vi "FPGA Definite Time Delay.vi"(0 "pick-up signal? (F)":bool, 1 "number of channels":T2=1 items=["1"=1, "2"=2, "3"=3, "4"=4, "5"=5, "6"=6, "7"=7, "8"=8, "9"=9, "10"=10, "11"=11, "12"=12, "13"=13, "14"=14, "15"=15, "16"=16], 5 "time delay settings":T1, 9 "input valid? (T)":bool=TRUE, 13 "instantaneous reset after tripping? (F)":bool) -> (4 "trip signal?":bool)   [LabVIEW 2013, in "NI_EP_Protection_FPGA.lvlib"]
doc: "Delays for the time interval that you specify in <B>time delay settings</B>, which includes the operate time and the reset time. Use this VI to build a protection relay with definite time delay characteristics, such as a 27 undervoltage relay, 50 instantaneous overcurrent relay, 59 overvoltage relay, and 81 frequency relay. You can compensate for the processing delay of the input energizing quantity to achieve higher operate time accuracy."
uses:
  <vilib>/addons/Electrical Power/Protection/NI_EP_Protection_FPGA.lvlib
  <vilib>/addons/Electrical Power/PQ/Resampling/FPGA/subVIs/fpga_NofCH.ctl
  <vilib>/addons/Electrical Power/Protection/Definite Time Delay/subVIs/fpga_Time Delay Cfg.ctl
  <vilib>/addons/Electrical Power/Protection/Definite Time Delay/subVIs/fpga_Feedback Var.ctl
  <vilib>/addons/Electrical Power/Protection/Definite Time Delay/subVIs/fpga_Timer Feedback Var.ctl
  <vilib>/addons/Electrical Power/Protection/Definite Time Delay/subVIs/fpga_State.ctl
  <vilib>/addons/Electrical Power/PQ/Resampling/NI_EP_Resample_FPGA.lvlib
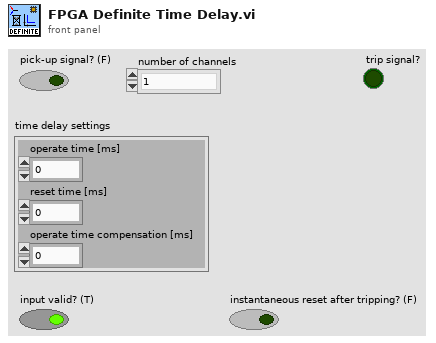
[diagram p1: front panel]
types:
  T1 = typedef "NI_EP_Protection_FPGA.lvlib/fpga_Time Delay Cfg.ctl" = cluster{"operate time [ms]":u32, "reset time [ms]":u32, "operate time compensation [ms]":u32}
  T2 = typedef "NI_EP_Resample_FPGA.lvlib/fpga_NofCH.ctl" = u8
  T3 = typedef "NI_EP_Protection_FPGA.lvlib/fpga_Feedback Var.ctl" = cluster{"timer":T4, "status":T5, "trip signal?":bool}
  T4 = typedef "NI_EP_Protection_FPGA.lvlib/fpga_Timer Feedback Var.ctl" = cluster{"time elapsed":u32, "start time of trip counting":u32, "start time of reseting":u32}
  T5 = typedef "NI_EP_Protection_FPGA.lvlib/fpga_State.ctl" = enum16{"Idle", "Trip Counting", "Tripped", "Reset Counting"}
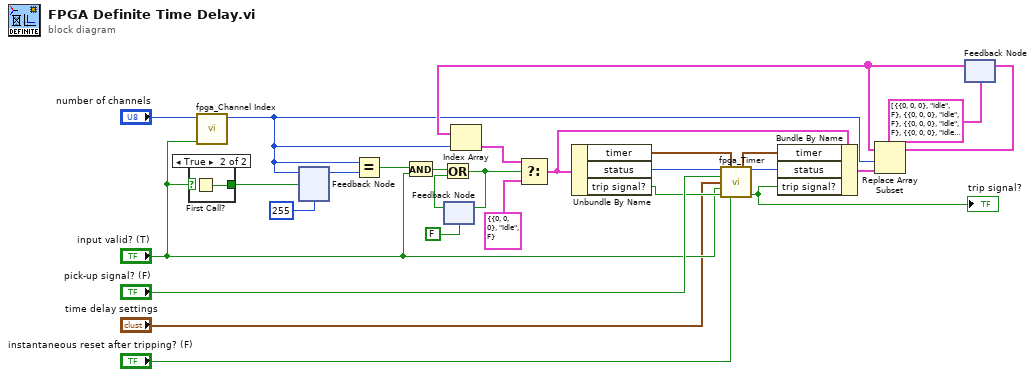
[diagram p0: block diagram]
diagram:
  n1 = case shown="True" "input valid? (T)" {
    selector: "input valid? (T)" -> [w28 _]
    tunnel: [w28 w29] -> w8
    frame False {
    }
    frame True {
      n2 = First Call?() -> (First Call?: T/F=w29:bool)
    }
  }
  n3 = call <vilib>:"fpga_Channel Index.vi"("input valid? (T)"="input valid? (T)", "number of channels"="number of channels") -> ("channel index"=w4:u8)  [unwired: 9 in]
  n4 = feedback #1(u8 255 ("channel index")) -> (w7:u8)
  n5 = feedback-in #1(w4, w8) -> ()
  n6 = Equal?(x=w4, y=w7) -> (x = y?=w11:bool)
  n7 = And(x=w11, y="input valid? (T)") -> (x .and. y?=w10:bool)
  n8 = feedback #2(FALSE) -> (w6:bool)
  n9 = Or(x=w10, y=w6) -> (x .or. y?=w19:bool)
  n10 = feedback-in #2(w19) -> ()
  n11 = feedback #3(T3[] [{"timer"={"time elapsed"=0, "start time of trip counting"=0, "start time of reseting"=0}, "status"=enum."Idle", "trip signal?"=FALSE}, {"timer"={"time elapsed"=0, "start time of trip counting"=0, "start time of reseting"=0}, "status"=enum."Idle", "trip signal?"=FALSE}, {"timer"={"time elapsed"=0, "start time of trip counting"=0, "start time of reseting"=0}, "status"=enum."Idle", "trip signal?"=FALSE}, {"timer"={"time elapsed"=0, "start time of trip counting"=0, "start time of reseting"=0}, "status"=enum."Idle", "trip signal?"=FALSE}, {"timer"={"time elapsed"=0, "start time of trip counting"=0, "start time of reseting"=0}, "status"=enum."Idle", "trip signal?"=FALSE}, {"timer"={"time elapsed"=0, "start time of trip counting"=0, "start time of reseting"=0}, "status"=enum."Idle", "trip signal?"=FALSE}, {"timer"={"time elapsed"=0, "start time of trip counting"=0, "start time of reseting"=0}, "status"=enum."Idle", "trip signal?"=FALSE}, {"timer"={"time elapsed"=0, "start time of trip counting"=0, "start time of reseting"=0}, "status"=enum."Idle", "trip signal?"=FALSE}, {"timer"={"time elapsed"=0, "start time of trip counting"=0, "start time of reseting"=0}, "status"=enum."Idle", "trip signal?"=FALSE}, {"timer"={"time elapsed"=0, "start time of trip counting"=0, "start time of reseting"=0}, "status"=enum."Idle", "trip signal?"=FALSE}, {"timer"={"time elapsed"=0, "start time of trip counting"=0, "start time of reseting"=0}, "status"=enum."Idle", "trip signal?"=FALSE}, {"timer"={"time elapsed"=0, "start time of trip counting"=0, "start time of reseting"=0}, "status"=enum."Idle", "trip signal?"=FALSE}, {"timer"={"time elapsed"=0, "start time of trip counting"=0, "start time of reseting"=0}, "status"=enum."Idle", "trip signal?"=FALSE}, {"timer"={"time elapsed"=0, "start time of trip counting"=0, "start time of reseting"=0}, "status"=enum."Idle", "trip signal?"=FALSE}, {"timer"={"time elapsed"=0, "start time of trip counting"=0, "start time of reseting"=0}, "status"=enum."Idle", "trip signal?"=FALSE}, {"timer"={"time elapsed"=0, "start time of trip counting"=0, "start time of reseting"=0}, "status"=enum."Idle", "trip signal?"=FALSE}] ("initialized array")) -> (w25:T3[])
  n12 = Index Array(array=w25, index=w4) -> (element=w22:T3)
  n13 = Select(t=w22, s=w19, f=T3 {"timer"={"time elapsed"=0, "start time of trip counting"=0, "start time of reseting"=0}, "status"=enum."Idle", "trip signal?"=FALSE} ("element")) -> (s? t:f=w12:T3)
  n14 = Unbundle By Name(w12) -> ("timer"=w23:T4, "status"=w15:T5, "trip signal?"=w14:bool)
  n15 = call <vilib>:"fpga_Timer.vi"("status in"=w15, "timing values in"=w23, "pick-up signal? (F)"="pick-up signal? (F)", "time delay settings"="time delay settings", "input valid?"="input valid? (T)", "trip signal in"=w14, "instantaneous reset after tripping? (F)"="instantaneous reset after tripping? (F)") -> ("timing values out"=w17:T4, "status out"=w16:T5, "trip signal out"=w26:bool)  [unwired: 6 in]
  "trip signal?" <- w26
  n16 = Bundle By Name(cluster=w12, "timer"=w17, "status"=w16, "trip signal?"=w26) -> (w24:T3)
  n17 = Replace Array Subset(array=w25, new element=w24, index=w4) -> (w13:T3[])
  n18 = feedback-in #3(w13) -> ()
